vi "getUnits.vi"(8 "error in (no error)":errorcluster, 11 "ACNET Device in":refnum<class "Copy of ACNET Device.lvclass">) -> (0 "error out":errorcluster, 2 "units":string, 3 "ACNET Device out":refnum<class "Copy of ACNET Device.lvclass">)   [LabVIEW 2013, in "Copy of ACNET Device.lvclass"]
uses:
  Copy of ACNET Device.lvclass
  Copy of ACNET Device.lvclass/Copy of ACNET Device.ctl
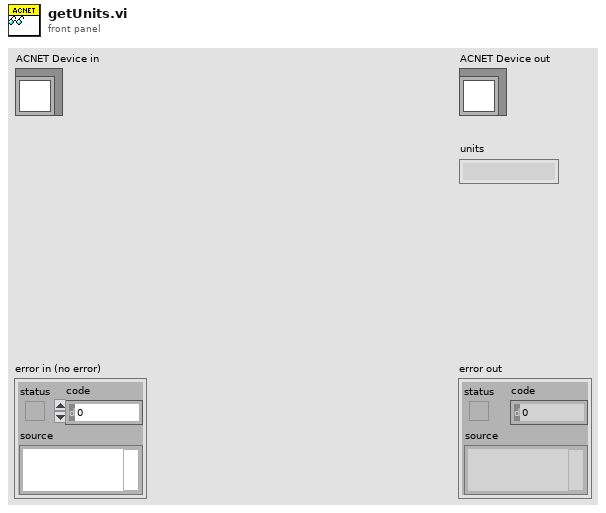
[diagram p1: front panel]
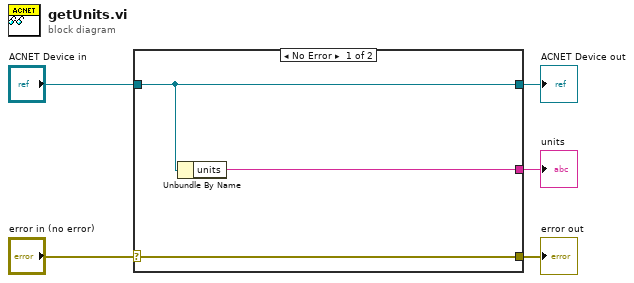
[diagram p0: block diagram]
diagram:
  n1 = case shown="No Error" "error in (no error)" {
    selector: "error in (no error)" -> [w8 w9]
    tunnel: [w8 w9] -> w4
    tunnel: [w7 w10] -> w2
    tunnel: "ACNET Device in" -> [w7 w10]
    tunnel: [w6 _] -> w1
    frame No Error {
      n2 = Unbundle By Name(w7) -> ("units"=w6:string)
    }
    frame Error {
    }
  }
  "error out" <- w4
  "ACNET Device out" <- w2
  "units" <- w1
